vi "generate sync struct.vi"(8 "error in (no error)":errorcluster, 11 "shared memory editor node in":refnum<class "module editor node.lvclass">) -> (0 "error out":errorcluster, 2 "struct string":string, 3 "shared memory editor node out":refnum<class "module editor node.lvclass">)   [LabVIEW 2014, in "Shared Memory editor node.lvclass"]
uses:
  Shared Memory editor node.lvclass
  <vilib>/NI/DCAF/Tag Editor Core/Configuration Editor/Classes/Module editor node/module editor node.lvclass
  cheddar/C Header Generator.lvlib
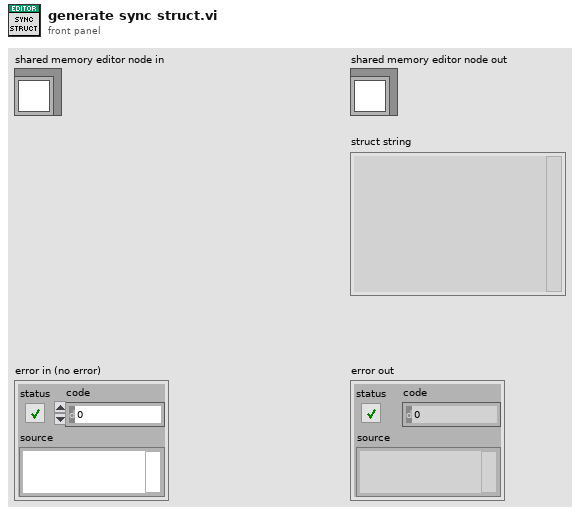
[diagram p1: front panel]
types:
  T1 = typedef "Shared Memory configuration.lvclass/sync item.ctl" = cluster{"mechanism":T2, "name":string}
  T2 = typedef "Shared Memory configuration.lvclass/sync mechanism.ctl" = enum16{"Semaphore"}
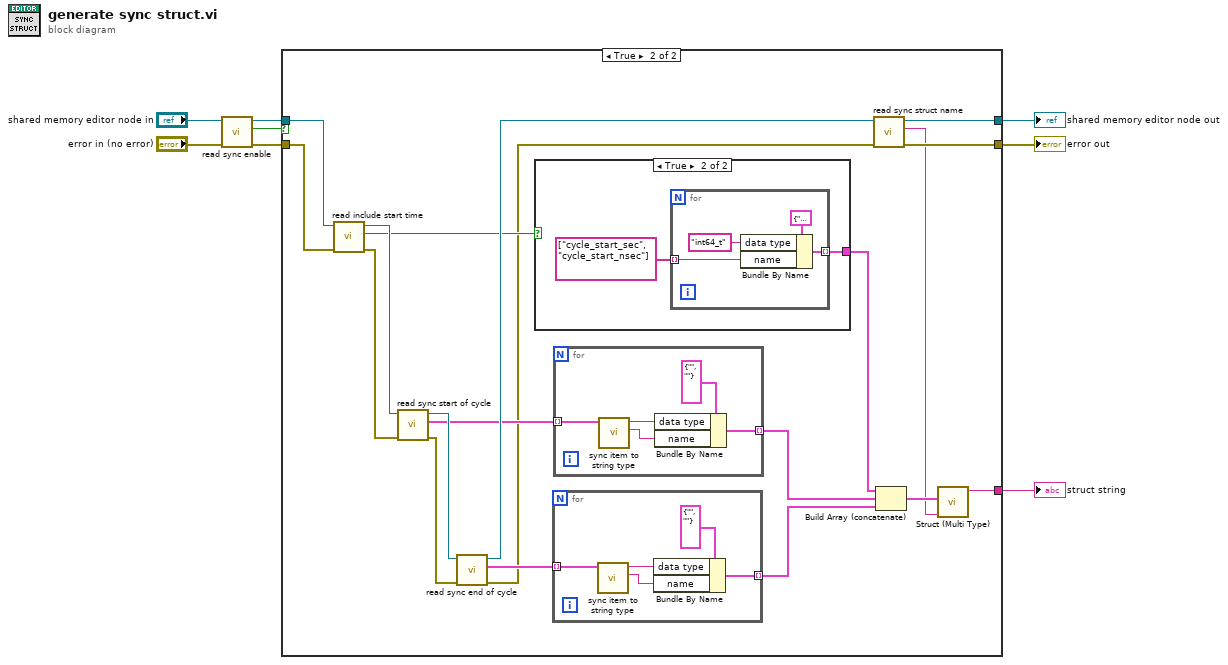
[diagram p0: block diagram]
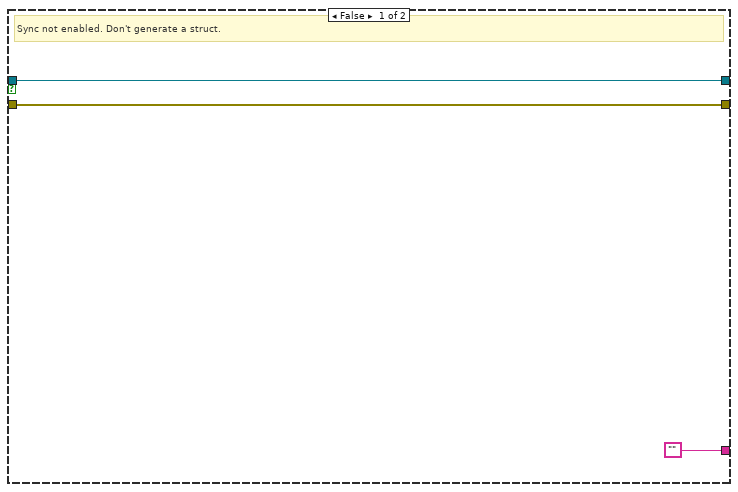
[diagram p2: hidden frame]
diagram:
  n1 = call "read sync enable.vi"("error in"="error in (no error)", "shared memory editor node"="shared memory editor node in") -> ("error out"=w5:errorcluster, "sync enable"=w7:bool, "shared memory editor node out"=w4:refnum<class "module editor node.lvclass">)  [unwired: 7 in]
  n2 = case shown="True" w7 {
    tunnel: w5 -> [w10 w20]
    tunnel: w4 -> [w11 w19]
    tunnel: [w11 w27] -> w3
    tunnel: [w10 w26] -> w1
    tunnel: ["" w23] -> w2
    frame False {
      # "Sync not enabled. Don't generate a struct."
    }
    frame True {
      n3 = call "read include start time.vi"("error in"=w20, "shared memory editor node"=w19) -> ("error out"=w18:errorcluster, "include start time"=w16:bool, "shared memory editor node out"=w17:refnum<class "module editor node.lvclass">)  [unwired: 7 in]
      n4 = call "read sync start of cycle.vi"("error in"=w18, "shared memory editor node"=w17) -> ("error out"=w29:errorcluster, "sync start of cycle"=w14:T1[], "shared memory editor node out"=w28:refnum<class "module editor node.lvclass">)  [unwired: 7 in]
      n5 = call "read sync end of cycle.vi"("error in"=w29, "shared memory editor node"=w28) -> ("error out"=w13:errorcluster, "sync end of cycle"=w15:T1[], "shared memory editor node out"=w21:refnum<class "module editor node.lvclass">)  [unwired: 7 in]
      n6 = case shown="True" w16 {
        tunnel: [_ w32] -> w22
        frame False {
        }
        frame True {
          n7 = for {
            tunnel: [w34] -> w32 mode=indexing
            tunnel: string[] ["cycle_start_sec", "cycle_start_nsec"] -> [w33] mode=indexing
            n8 = Bundle By Name(cluster=cluster{"data type":string, "name":string} {"data type"="", "name"=""} ("Variable"), "data type"="int64_t", "name"=w33) -> (w34:cluster{"data type":string, "name":string})
          }
        }
      }
      n9 = for {
        tunnel: w15 -> [w38] mode=indexing
        tunnel: [w37] -> w12 mode=indexing
        n10 = call "sync item to string type.vi"("sync item"=w38) -> ("variable name"=w39:string, "variable type"=w40:string)  [unwired: 9 in]
        n11 = Bundle By Name(cluster=cluster{"data type":string, "name":string} {"data type"="", "name"=""} ("Variable"), "data type"=w40, "name"=w39) -> (w37:cluster{"data type":string, "name":string})
      }
      n12 = for {
        tunnel: w14 -> [w43] mode=indexing
        tunnel: [w42] -> w30 mode=indexing
        n13 = call "sync item to string type.vi"("sync item"=w43) -> ("variable name"=w44:string, "variable type"=w45:string)  [unwired: 9 in]
        n14 = Bundle By Name(cluster=cluster{"data type":string, "name":string} {"data type"="", "name"=""} ("Variable"), "data type"=w45, "name"=w44) -> (w42:cluster{"data type":string, "name":string})
      }
      n15 = call "read sync struct name.vi"("error in"=w13, "shared memory editor node"=w21) -> ("error out"=w26:errorcluster, "sync struct name"=w24:string, "shared memory editor node out"=w27:refnum<class "module editor node.lvclass">)  [unwired: 7 in]
      n16 = Build Array (concatenate)(w22, w30, w12) -> (w25:cluster{"data type":string, "name":string}[])
      n17 = call "Struct (Multi Type).vi"("Struct name"=w24, "Variables"=w25) -> ("String out"=w23:string)  [unwired: 9 in]
    }
  }
  "shared memory editor node out" <- w3
  "error out" <- w1
  "struct string" <- w2
